vi "Thev-Fq to L.vi"(1 "Fq (Hz)":dbl) -> (0 "L (mm)":dbl)   [LabVIEW 2015]
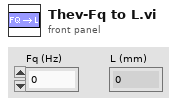
[diagram p1: front panel]
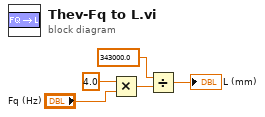
[diagram p0: block diagram]
diagram:
  n1 = Multiply(x=4.0, y="Fq (Hz)") -> (x*y=w3:dbl)
  n2 = Divide(x=343000.0, y=w3) -> (x/y=→"L (mm)":dbl)
